vi "X and Y Coordinate Polar.vi"(8 "Rc":u32, 9 "Yc":u32, 10 "Xc":u32, 11 "Selected Coordinate":T1(ring)) -> (1 "X,Y selected":T1(ring), 2 "Youtput":u32, 3 "Xoutput":u32)   [LabVIEW 2020]
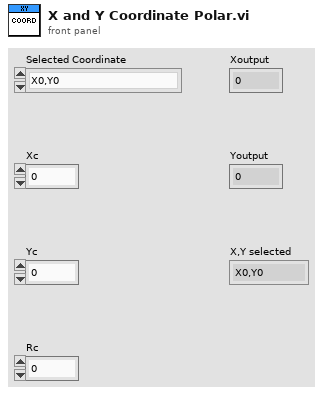
[diagram p1: front panel]
types:
  T1 = enum16{"X0,Y0", "X1,Y1", "X2,Y2", "X3,Y3", "X4,Y4", "X5,Y5", "X6,Y6", "X7,Y7", "X8,Y8", "X9,Y9", "X10,Y10", "X11,Y11", "X12,Y12", "X13,Y13", "X14,Y14", "X15,Y15", "X16,Y16", "X17,Y17", "X18,Y18", "X19,Y19", "X20,Y20", "X21,Y21", "X22,Y22", "X23,Y23"}
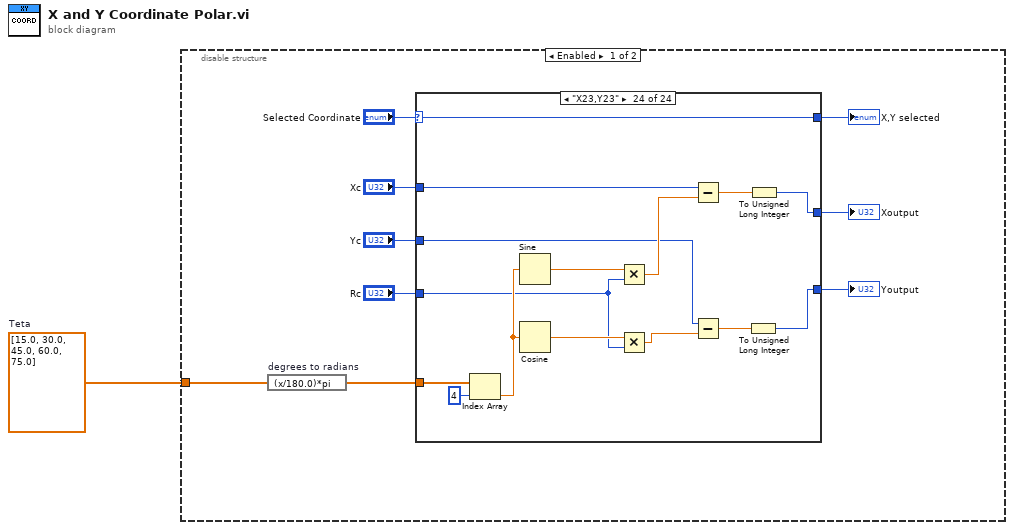
[diagram p0: block diagram]
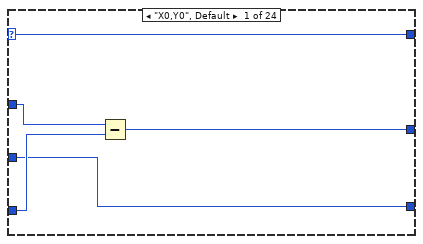
[diagram p2: hidden frame]
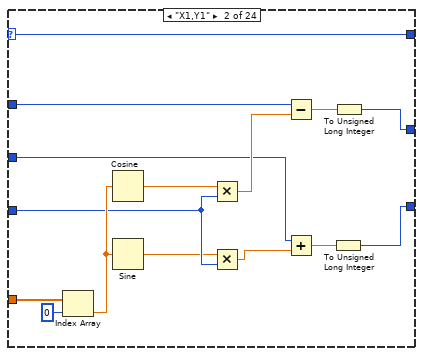
[diagram p3: hidden frame]
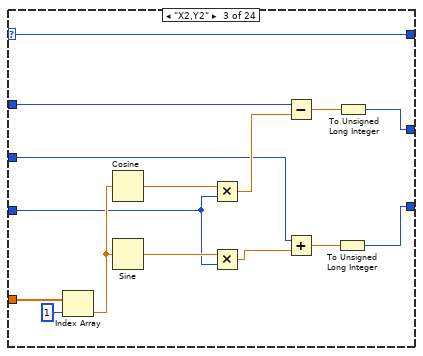
[diagram p4: hidden frame]
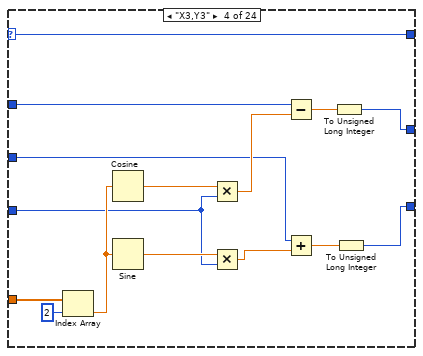
[diagram p5: hidden frame]
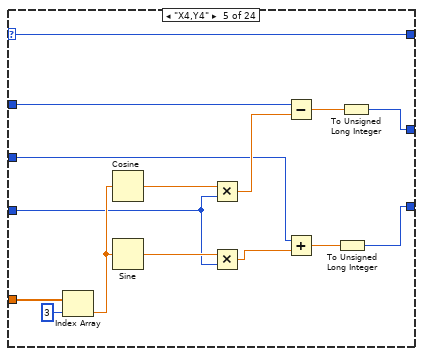
[diagram p6: hidden frame]
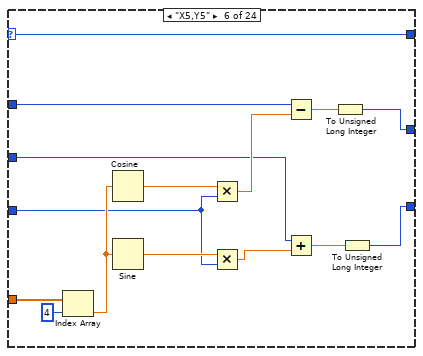
[diagram p7: hidden frame]
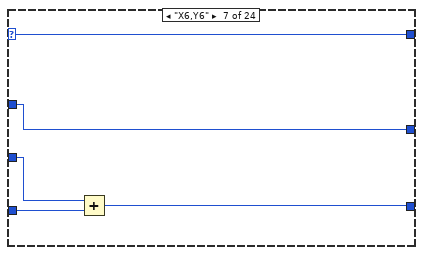
[diagram p8: hidden frame]
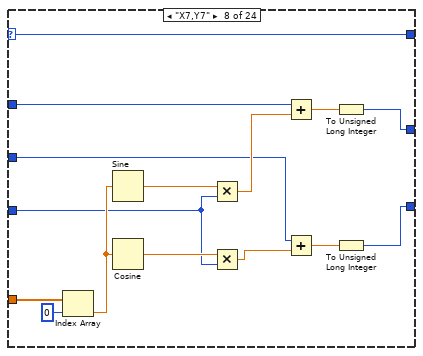
[diagram p9: hidden frame]
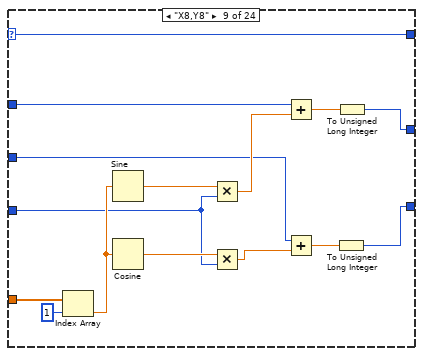
[diagram p10: hidden frame]
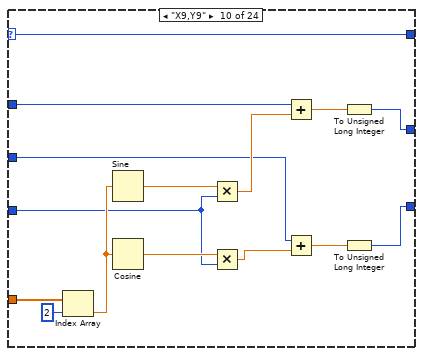
[diagram p11: hidden frame]
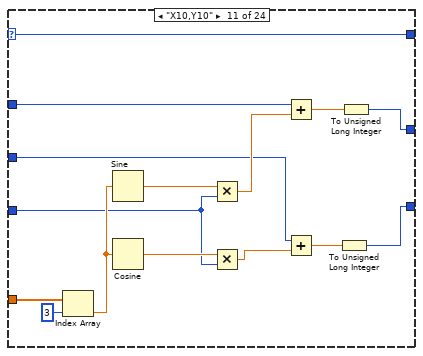
[diagram p12: hidden frame]
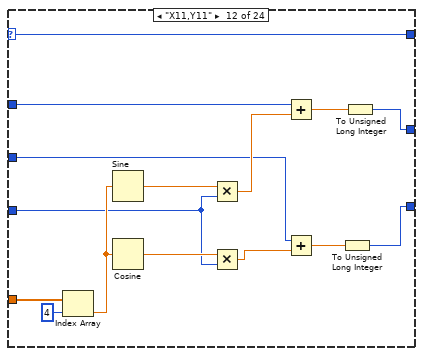
[diagram p13: hidden frame]
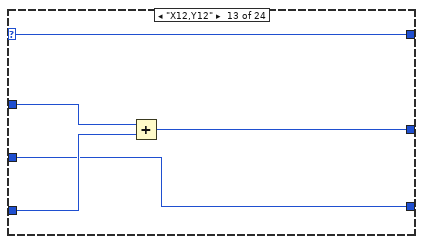
[diagram p14: hidden frame]
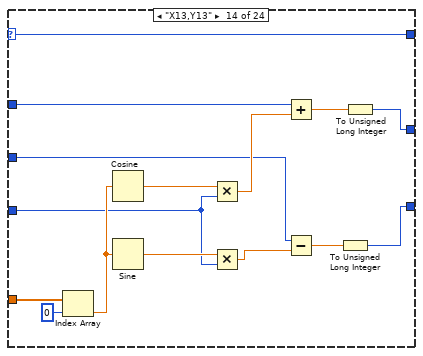
[diagram p15: hidden frame]
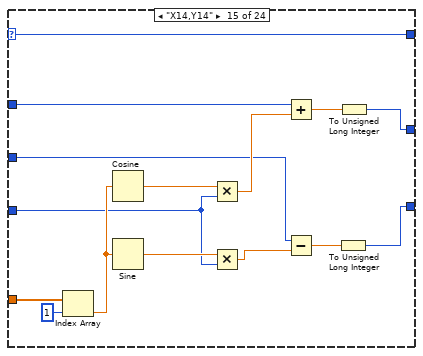
[diagram p16: hidden frame]
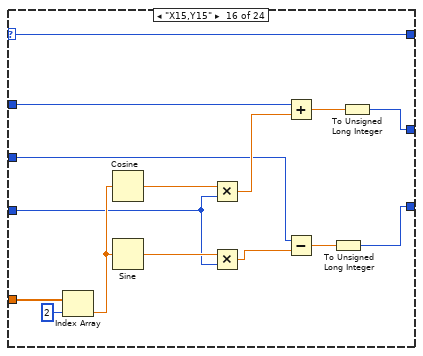
[diagram p17: hidden frame]
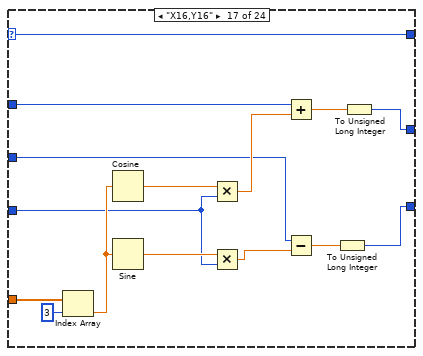
[diagram p18: hidden frame]
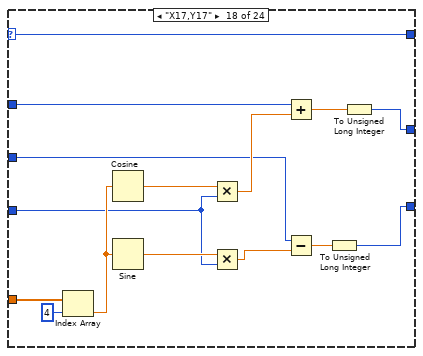
[diagram p19: hidden frame]
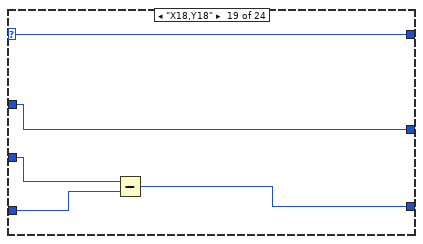
[diagram p20: hidden frame]
diagram:
  w1 = dbl[] [15.0, 30.0, 45.0, 60.0, 75.0]  # Teta
  n1 = disable-structure shown="Enabled" {
    disable-tunnel: w1 -> [w3 w331]
    frame Enabled {
      n2 = expression code="(x/180.0)*pi" "degrees to radians"(w3) -> (w2:dbl[])
      n3 = case shown="\"X23,Y23\"" "Selected Coordinate" {
        selector: "Selected Coordinate" -> [w15 w30 w45 w60 w75 w90 w91 w110 w125 w140 w155 w170 w171 w190 w205 w220 w235 w250 w254 w270 w285 w300 w315 w330]
        tunnel: [w15 w30 w45 w60 w75 w90 w91 w110 w125 w140 w155 w170 w171 w190 w205 w220 w235 w250 w254 w270 w285 w300 w315 w330] -> w9
        tunnel: "Xc" -> [w14 w29 w44 w59 w74 w89 w95 w109 w124 w139 w154 w169 w175 w189 w204 w219 w234 w249 w255 w269 w284 w299 w314 w329]
        tunnel: "Rc" -> [w13 w23 w36 w51 w66 w81 w93 w101 w116 w131 w146 w161 w174 w181 w196 w211 w226 w241 w252 w261 w276 w291 w306 w321]
        tunnel: [w12 w17 w32 w47 w62 w77 w95 w97 w112 w127 w142 w157 w173 w177 w192 w207 w222 w237 w255 w257 w272 w287 w302 w317] -> w6
        tunnel: "Yc" -> [w11 w22 w35 w50 w65 w80 w94 w100 w115 w130 w145 w160 w172 w180 w195 w210 w225 w240 w253 w260 w275 w290 w305 w320]
        tunnel: [w11 w16 w31 w46 w61 w76 w92 w96 w111 w126 w141 w156 w172 w176 w191 w206 w221 w236 w251 w256 w271 w286 w301 w316] -> w4
        tunnel: w2 -> [_ w28 w43 w58 w73 w88 _ w108 w123 w138 w153 w168 _ w188 w203 w218 w233 w248 _ w268 w283 w298 w313 w328]
        frame "X0,Y0", Default {
          n4 = Subtract(x=w14, y=w13) -> (x-y=w12:u32)
        }
        frame "X1,Y1" {
          n5 = Index Array(array=w28, index=0) -> (element=w24:dbl)
          n6 = Cosine(x=w24) -> (cos(x)=w19:dbl)
          n7 = Sine(x=w24) -> (sin(x)=w18:dbl)
          n8 = Multiply(x=w19, y=w23) -> (x*y=w26:dbl)
          n9 = Multiply(x=w18, y=w23) -> (x*y=w21:dbl)
          n10 = Subtract(x=w29, y=w26) -> (x-y=w25:dbl)
          n11 = Add(x=w22, y=w21) -> (x+y=w20:dbl)
          n12 = To Unsigned Long Integer(number=w20) -> (unsigned 32bit integer=w16:u32)
          n13 = To Unsigned Long Integer(number=w25) -> (unsigned 32bit integer=w17:u32)
        }
        frame "X2,Y2" {
          n14 = Index Array(array=w43, index=1) -> (element=w38:dbl)
          n15 = Cosine(x=w38) -> (cos(x)=w41:dbl)
          n16 = Sine(x=w38) -> (sin(x)=w37:dbl)
          n17 = Multiply(x=w41, y=w36) -> (x*y=w40:dbl)
          n18 = Multiply(x=w37, y=w36) -> (x*y=w34:dbl)
          n19 = Subtract(x=w44, y=w40) -> (x-y=w39:dbl)
          n20 = Add(x=w35, y=w34) -> (x+y=w33:dbl)
          n21 = To Unsigned Long Integer(number=w33) -> (unsigned 32bit integer=w31:u32)
          n22 = To Unsigned Long Integer(number=w39) -> (unsigned 32bit integer=w32:u32)
        }
        frame "X3,Y3" {
          n23 = Index Array(array=w58, index=2) -> (element=w53:dbl)
          n24 = Cosine(x=w53) -> (cos(x)=w56:dbl)
          n25 = Sine(x=w53) -> (sin(x)=w52:dbl)
          n26 = Multiply(x=w56, y=w51) -> (x*y=w55:dbl)
          n27 = Multiply(x=w52, y=w51) -> (x*y=w49:dbl)
          n28 = Subtract(x=w59, y=w55) -> (x-y=w54:dbl)
          n29 = Add(x=w50, y=w49) -> (x+y=w48:dbl)
          n30 = To Unsigned Long Integer(number=w54) -> (unsigned 32bit integer=w47:u32)
          n31 = To Unsigned Long Integer(number=w48) -> (unsigned 32bit integer=w46:u32)
        }
        frame "X4,Y4" {
          n32 = Index Array(array=w73, index=3) -> (element=w68:dbl)
          n33 = Cosine(x=w68) -> (cos(x)=w71:dbl)
          n34 = Sine(x=w68) -> (sin(x)=w67:dbl)
          n35 = Multiply(x=w71, y=w66) -> (x*y=w70:dbl)
          n36 = Multiply(x=w67, y=w66) -> (x*y=w64:dbl)
          n37 = Subtract(x=w74, y=w70) -> (x-y=w69:dbl)
          n38 = Add(x=w65, y=w64) -> (x+y=w63:dbl)
          n39 = To Unsigned Long Integer(number=w63) -> (unsigned 32bit integer=w61:u32)
          n40 = To Unsigned Long Integer(number=w69) -> (unsigned 32bit integer=w62:u32)
        }
        frame "X5,Y5" {
          n41 = Index Array(array=w88, index=4) -> (element=w83:dbl)
          n42 = Cosine(x=w83) -> (cos(x)=w86:dbl)
          n43 = Sine(x=w83) -> (sin(x)=w82:dbl)
          n44 = Multiply(x=w86, y=w81) -> (x*y=w85:dbl)
          n45 = Multiply(x=w82, y=w81) -> (x*y=w79:dbl)
          n46 = Subtract(x=w89, y=w85) -> (x-y=w84:dbl)
          n47 = Add(x=w80, y=w79) -> (x+y=w78:dbl)
          n48 = To Unsigned Long Integer(number=w84) -> (unsigned 32bit integer=w77:u32)
          n49 = To Unsigned Long Integer(number=w78) -> (unsigned 32bit integer=w76:u32)
        }
        frame "X6,Y6" {
          n50 = Add(x=w94, y=w93) -> (x+y=w92:u32)
        }
        frame "X7,Y7" {
          n51 = Index Array(array=w108, index=0) -> (element=w103:dbl)
          n52 = Sine(x=w103) -> (sin(x)=w106:dbl)
          n53 = Cosine(x=w103) -> (cos(x)=w102:dbl)
          n54 = Multiply(x=w106, y=w101) -> (x*y=w105:dbl)
          n55 = Multiply(x=w102, y=w101) -> (x*y=w99:dbl)
          n56 = Add(x=w109, y=w105) -> (x+y=w104:dbl)
          n57 = Add(x=w100, y=w99) -> (x+y=w98:dbl)
          n58 = To Unsigned Long Integer(number=w104) -> (unsigned 32bit integer=w97:u32)
          n59 = To Unsigned Long Integer(number=w98) -> (unsigned 32bit integer=w96:u32)
        }
        frame "X8,Y8" {
          n60 = Index Array(array=w123, index=1) -> (element=w118:dbl)
          n61 = Sine(x=w118) -> (sin(x)=w121:dbl)
          n62 = Cosine(x=w118) -> (cos(x)=w117:dbl)
          n63 = Multiply(x=w121, y=w116) -> (x*y=w120:dbl)
          n64 = Multiply(x=w117, y=w116) -> (x*y=w114:dbl)
          n65 = Add(x=w124, y=w120) -> (x+y=w119:dbl)
          n66 = Add(x=w115, y=w114) -> (x+y=w113:dbl)
          n67 = To Unsigned Long Integer(number=w113) -> (unsigned 32bit integer=w111:u32)
          n68 = To Unsigned Long Integer(number=w119) -> (unsigned 32bit integer=w112:u32)
        }
        frame "X9,Y9" {
          n69 = Index Array(array=w138, index=2) -> (element=w133:dbl)
          n70 = Sine(x=w133) -> (sin(x)=w136:dbl)
          n71 = Cosine(x=w133) -> (cos(x)=w132:dbl)
          n72 = Multiply(x=w136, y=w131) -> (x*y=w135:dbl)
          n73 = Multiply(x=w132, y=w131) -> (x*y=w129:dbl)
          n74 = Add(x=w139, y=w135) -> (x+y=w134:dbl)
          n75 = Add(x=w130, y=w129) -> (x+y=w128:dbl)
          n76 = To Unsigned Long Integer(number=w134) -> (unsigned 32bit integer=w127:u32)
          n77 = To Unsigned Long Integer(number=w128) -> (unsigned 32bit integer=w126:u32)
        }
        frame "X10,Y10" {
          n78 = Index Array(array=w153, index=3) -> (element=w148:dbl)
          n79 = Sine(x=w148) -> (sin(x)=w151:dbl)
          n80 = Cosine(x=w148) -> (cos(x)=w147:dbl)
          n81 = Multiply(x=w151, y=w146) -> (x*y=w150:dbl)
          n82 = Multiply(x=w147, y=w146) -> (x*y=w144:dbl)
          n83 = Add(x=w154, y=w150) -> (x+y=w149:dbl)
          n84 = Add(x=w145, y=w144) -> (x+y=w143:dbl)
          n85 = To Unsigned Long Integer(number=w143) -> (unsigned 32bit integer=w141:u32)
          n86 = To Unsigned Long Integer(number=w149) -> (unsigned 32bit integer=w142:u32)
        }
        frame "X11,Y11" {
          n87 = Index Array(array=w168, index=4) -> (element=w163:dbl)
          n88 = Sine(x=w163) -> (sin(x)=w166:dbl)
          n89 = Cosine(x=w163) -> (cos(x)=w162:dbl)
          n90 = Multiply(x=w166, y=w161) -> (x*y=w165:dbl)
          n91 = Multiply(x=w162, y=w161) -> (x*y=w159:dbl)
          n92 = Add(x=w169, y=w165) -> (x+y=w164:dbl)
          n93 = Add(x=w160, y=w159) -> (x+y=w158:dbl)
          n94 = To Unsigned Long Integer(number=w158) -> (unsigned 32bit integer=w156:u32)
          n95 = To Unsigned Long Integer(number=w164) -> (unsigned 32bit integer=w157:u32)
        }
        frame "X12,Y12" {
          n96 = Add(x=w175, y=w174) -> (x+y=w173:u32)
        }
        frame "X13,Y13" {
          n97 = Index Array(array=w188, index=0) -> (element=w183:dbl)
          n98 = Cosine(x=w183) -> (cos(x)=w186:dbl)
          n99 = Sine(x=w183) -> (sin(x)=w182:dbl)
          n100 = Multiply(x=w186, y=w181) -> (x*y=w185:dbl)
          n101 = Multiply(x=w182, y=w181) -> (x*y=w179:dbl)
          n102 = Add(x=w189, y=w185) -> (x+y=w184:dbl)
          n103 = Subtract(x=w180, y=w179) -> (x-y=w178:dbl)
          n104 = To Unsigned Long Integer(number=w178) -> (unsigned 32bit integer=w176:u32)
          n105 = To Unsigned Long Integer(number=w184) -> (unsigned 32bit integer=w177:u32)
        }
        frame "X14,Y14" {
          n106 = Index Array(array=w203, index=1) -> (element=w198:dbl)
          n107 = Cosine(x=w198) -> (cos(x)=w201:dbl)
          n108 = Sine(x=w198) -> (sin(x)=w197:dbl)
          n109 = Multiply(x=w201, y=w196) -> (x*y=w200:dbl)
          n110 = Multiply(x=w197, y=w196) -> (x*y=w194:dbl)
          n111 = Add(x=w204, y=w200) -> (x+y=w199:dbl)
          n112 = Subtract(x=w195, y=w194) -> (x-y=w193:dbl)
          n113 = To Unsigned Long Integer(number=w193) -> (unsigned 32bit integer=w191:u32)
          n114 = To Unsigned Long Integer(number=w199) -> (unsigned 32bit integer=w192:u32)
        }
        frame "X15,Y15" {
          n115 = Index Array(array=w218, index=2) -> (element=w213:dbl)
          n116 = Cosine(x=w213) -> (cos(x)=w216:dbl)
          n117 = Sine(x=w213) -> (sin(x)=w212:dbl)
          n118 = Multiply(x=w216, y=w211) -> (x*y=w215:dbl)
          n119 = Multiply(x=w212, y=w211) -> (x*y=w209:dbl)
          n120 = Add(x=w219, y=w215) -> (x+y=w214:dbl)
          n121 = Subtract(x=w210, y=w209) -> (x-y=w208:dbl)
          n122 = To Unsigned Long Integer(number=w208) -> (unsigned 32bit integer=w206:u32)
          n123 = To Unsigned Long Integer(number=w214) -> (unsigned 32bit integer=w207:u32)
        }
        frame "X16,Y16" {
          n124 = Index Array(array=w233, index=3) -> (element=w228:dbl)
          n125 = Cosine(x=w228) -> (cos(x)=w231:dbl)
          n126 = Sine(x=w228) -> (sin(x)=w227:dbl)
          n127 = Multiply(x=w231, y=w226) -> (x*y=w230:dbl)
          n128 = Multiply(x=w227, y=w226) -> (x*y=w224:dbl)
          n129 = Add(x=w234, y=w230) -> (x+y=w229:dbl)
          n130 = Subtract(x=w225, y=w224) -> (x-y=w223:dbl)
          n131 = To Unsigned Long Integer(number=w223) -> (unsigned 32bit integer=w221:u32)
          n132 = To Unsigned Long Integer(number=w229) -> (unsigned 32bit integer=w222:u32)
        }
        frame "X17,Y17" {
          n133 = Index Array(array=w248, index=4) -> (element=w243:dbl)
          n134 = Cosine(x=w243) -> (cos(x)=w246:dbl)
          n135 = Sine(x=w243) -> (sin(x)=w242:dbl)
          n136 = Multiply(x=w246, y=w241) -> (x*y=w245:dbl)
          n137 = Multiply(x=w242, y=w241) -> (x*y=w239:dbl)
          n138 = Add(x=w249, y=w245) -> (x+y=w244:dbl)
          n139 = Subtract(x=w240, y=w239) -> (x-y=w238:dbl)
          n140 = To Unsigned Long Integer(number=w238) -> (unsigned 32bit integer=w236:u32)
          n141 = To Unsigned Long Integer(number=w244) -> (unsigned 32bit integer=w237:u32)
        }
        frame "X18,Y18" {
          n142 = Subtract(x=w253, y=w252) -> (x-y=w251:u32)
        }
        frame "X19,Y19" {
          n143 = Index Array(array=w268, index=0) -> (element=w263:dbl)
          n144 = Sine(x=w263) -> (sin(x)=w266:dbl)
          n145 = Cosine(x=w263) -> (cos(x)=w262:dbl)
          n146 = Multiply(x=w266, y=w261) -> (x*y=w265:dbl)
          n147 = Multiply(x=w262, y=w261) -> (x*y=w259:dbl)
          n148 = Subtract(x=w269, y=w265) -> (x-y=w264:dbl)
          n149 = Subtract(x=w260, y=w259) -> (x-y=w258:dbl)
          n150 = To Unsigned Long Integer(number=w264) -> (unsigned 32bit integer=w257:u32)
          n151 = To Unsigned Long Integer(number=w258) -> (unsigned 32bit integer=w256:u32)
        }
        frame "X20,Y20" {
          n152 = Index Array(array=w283, index=1) -> (element=w278:dbl)
          n153 = Sine(x=w278) -> (sin(x)=w281:dbl)
          n154 = Cosine(x=w278) -> (cos(x)=w277:dbl)
          n155 = Multiply(x=w281, y=w276) -> (x*y=w280:dbl)
          n156 = Multiply(x=w277, y=w276) -> (x*y=w274:dbl)
          n157 = Subtract(x=w284, y=w280) -> (x-y=w279:dbl)
          n158 = Subtract(x=w275, y=w274) -> (x-y=w273:dbl)
          n159 = To Unsigned Long Integer(number=w273) -> (unsigned 32bit integer=w271:u32)
          n160 = To Unsigned Long Integer(number=w279) -> (unsigned 32bit integer=w272:u32)
        }
        frame "X21,Y21" {
          n161 = Index Array(array=w298, index=2) -> (element=w293:dbl)
          n162 = Sine(x=w293) -> (sin(x)=w296:dbl)
          n163 = Cosine(x=w293) -> (cos(x)=w292:dbl)
          n164 = Multiply(x=w296, y=w291) -> (x*y=w295:dbl)
          n165 = Multiply(x=w292, y=w291) -> (x*y=w289:dbl)
          n166 = Subtract(x=w299, y=w295) -> (x-y=w294:dbl)
          n167 = Subtract(x=w290, y=w289) -> (x-y=w288:dbl)
          n168 = To Unsigned Long Integer(number=w294) -> (unsigned 32bit integer=w287:u32)
          n169 = To Unsigned Long Integer(number=w288) -> (unsigned 32bit integer=w286:u32)
        }
        frame "X22,Y22" {
          n170 = Index Array(array=w313, index=3) -> (element=w308:dbl)
          n171 = Sine(x=w308) -> (sin(x)=w311:dbl)
          n172 = Cosine(x=w308) -> (cos(x)=w307:dbl)
          n173 = Multiply(x=w311, y=w306) -> (x*y=w310:dbl)
          n174 = Multiply(x=w307, y=w306) -> (x*y=w304:dbl)
          n175 = Subtract(x=w314, y=w310) -> (x-y=w309:dbl)
          n176 = Subtract(x=w305, y=w304) -> (x-y=w303:dbl)
          n177 = To Unsigned Long Integer(number=w303) -> (unsigned 32bit integer=w301:u32)
          n178 = To Unsigned Long Integer(number=w309) -> (unsigned 32bit integer=w302:u32)
        }
        frame "X23,Y23" {
          n179 = Index Array(array=w328, index=4) -> (element=w323:dbl)
          n180 = Sine(x=w323) -> (sin(x)=w326:dbl)
          n181 = Cosine(x=w323) -> (cos(x)=w322:dbl)
          n182 = Multiply(x=w326, y=w321) -> (x*y=w325:dbl)
          n183 = Multiply(x=w322, y=w321) -> (x*y=w319:dbl)
          n184 = Subtract(x=w329, y=w325) -> (x-y=w324:dbl)
          n185 = Subtract(x=w320, y=w319) -> (x-y=w318:dbl)
          n186 = To Unsigned Long Integer(number=w318) -> (unsigned 32bit integer=w316:u32)
          n187 = To Unsigned Long Integer(number=w324) -> (unsigned 32bit integer=w317:u32)
        }
      }
      "Xoutput" <- w6
      "Youtput" <- w4
      "X,Y selected" <- w9
    }
    frame Disabled {
      n188 = Index Array(array=w331, index=0) -> (element=w333:dbl)
      n189 = expression code="(x/180.0)*pi" "degrees to radians"(w333) -> (w332:dbl)
      n190 = Cosine(x=w332) -> ()  [unwired: 1 out]
    }
  }
